vi "Publish Test Value.vi"(8 "error in (no error)":errorcluster, 11 "RootModelPublishesDoubleFloatX in":refnum<class "RootModelPublishesDoubleFloatX.lvclass">) -> (0 "error out":errorcluster, 3 "RootModelPublishesDoubleFloatX out":refnum<class "RootModelPublishesDoubleFloatX.lvclass">)   [LabVIEW 2020, in "RootModelPublishesDoubleFloatX.lvlib" / "RootModelPublishesDoubleFloatX.lvclass"]
uses:
  RootModelPublishesDoubleFloatX.lvclass
  RootModelPublishesDoubleFloatX.lvclass/RootModelPublishesDoubleFloatX.ctl
  Source/IModel/IModel/IModel.lvclass
  C:/Git/mva-core/Source/RootModel/RootModel/RootModel.lvclass
  C:/Git/mva-core/Source/IModel/IModel/IModel.lvclass
  C:/Git/mva-core/Source/IObserver/IObserver/IObserver.lvclass
  C:/Program Files (x86)/National Instruments/LabVIEW 2020/vi.lib/ActorFramework/Actor/Actor.lvclass
  C:/Git/mva-core/Test/Doubles/RootModelPublishesDoubleFloatX/RootModelPublishesDoubleFloatX.lvclass
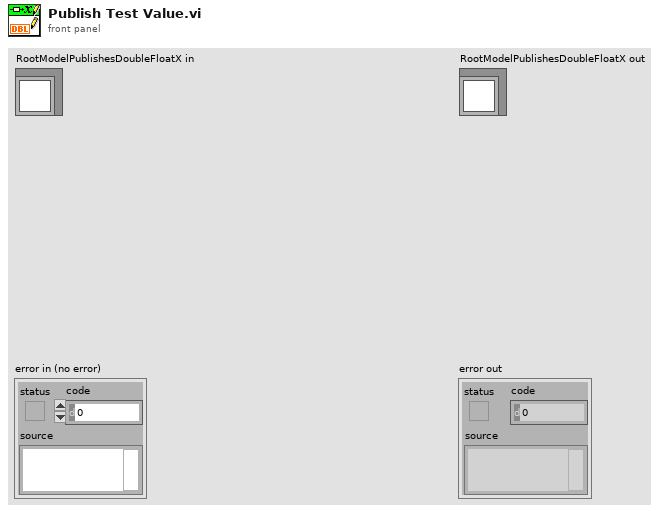
[diagram p1: front panel]
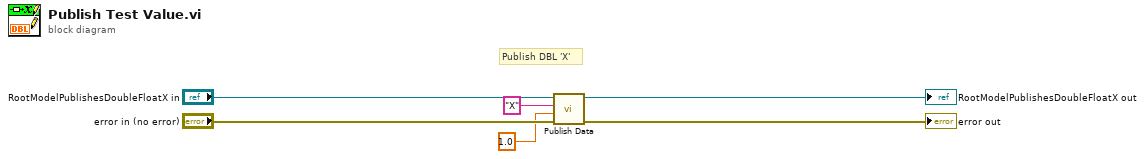
[diagram p0: block diagram]
diagram:
  # "Publish DBL 'X'"
  n1 = call "Publish Data.vi"("error in (no error)"="error in (no error)", "Data to Publish"=1.0, "Datum Name"="X", "IModel in"="RootModelPublishesDoubleFloatX in") -> ("error out"=→"error out":errorcluster, "IModel out"=→"RootModelPublishesDoubleFloatX out":refnum<class "RootModelPublishesDoubleFloatX.lvclass">)  [unwired: 6 in]
